vi "Get SMO Public API.vi"(8 "error in (no error)":errorcluster, 11 "Instrument.Example In":refnum<class "Instrument.OxfordVRM.lvclass">) -> (0 "error out":errorcluster, 2 "Commands":string[](array[string]), 3 "Instrument.Example out":refnum<class "Instrument.OxfordVRM.lvclass">)   [LabVIEW 2016, in "Instrument.OxfordVRM.lvclass"]
uses:
  Instrument.OxfordVRM.lvclass
  Typedefs/Instrument.Oxford1820.Commands-enum.ctl
  <userlib>/LevyLab/Levylab Instruments/Instrument Types/Cryostat/Instrument.Cryostat.lvclass
panel:
  in  "Commands":T1
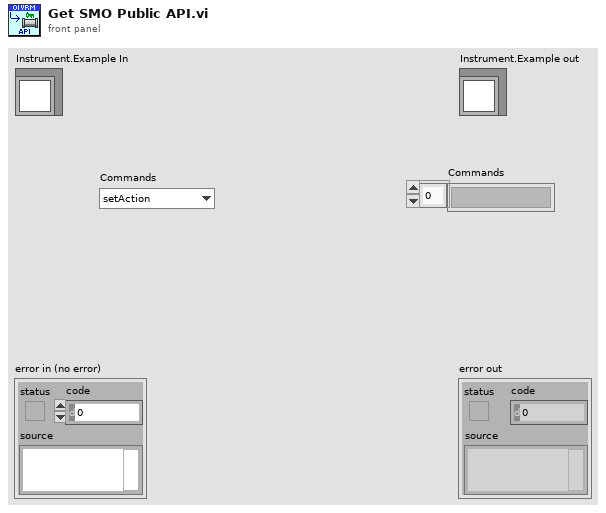
[diagram p1: front panel]
types:
  T1 = typedef "Instrument.OxfordVRM.lvclass/Instrument.Oxford1820.Commands-enum.ctl" = enum16{"setAction", "setTarget", "setSwitchHeat", "setLambda", "setFillMode", "setNeedleValve", "setMagnetField", "getStatus", "getTarget", "getSwitchHeat", "getPSUField", "newcommand", "getMagnetField"}
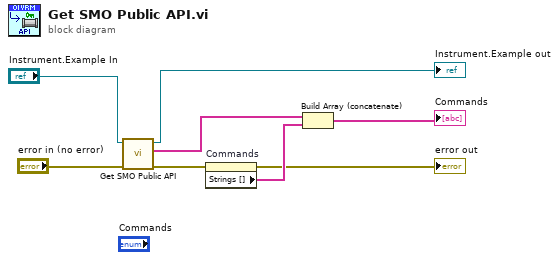
[diagram p0: block diagram]
diagram:
  n1 = call-parent "Get SMO Public API.vi"("error in (no error)"="error in (no error)", "Instrument in"="Instrument.Example In") -> ("error out"=w2:errorcluster, "Commands"=w5:string[], "Instrument out"=→"Instrument.Example out":refnum<class "Instrument.OxfordVRM.lvclass">)  [unwired: 7 in]
  n2 = property on="Commands" class="Enum (strict)"(error in=w2) -> (error out=→"error out":errorcluster, "Strings []"=w3:string[])  [unwired: 1 in, 1 out]
  n3 = Build Array (concatenate)(w5, w3) -> (→"Commands":string[])
